vi "COMANDOS_QUIZ1.vi"() -> ()   [LabVIEW 2017]
panel:
  out "comentarios":string[](array[string])
  out "cmd users":string[](array[string])
  out "OP PRINCIPALES":T1(ring)
  out "CONFIG LED":T2(ring)
  out "CONFIG BOTON":T2(ring)
  out "L 3":string
  out "L 2":string
  out "L 1":string
  out "B 3":string
  out "B 2":string
  out "B 1":string
  out "time":u32
  out "contador":i32
  in  "TRAMA DE PRUEBA":string
  in  "BOTÓN 3":bool
  in  "BOTÓN 2":bool
  in  "BOTÓN 1":bool
  out "LED 3":bool
  out "LED 2":bool
  out "LED 1":bool
  out "at+<cmd>?response":string[](array[string])
  in  "stop":bool
  in  "send":bool
  out "Out":string
  in  "In":string
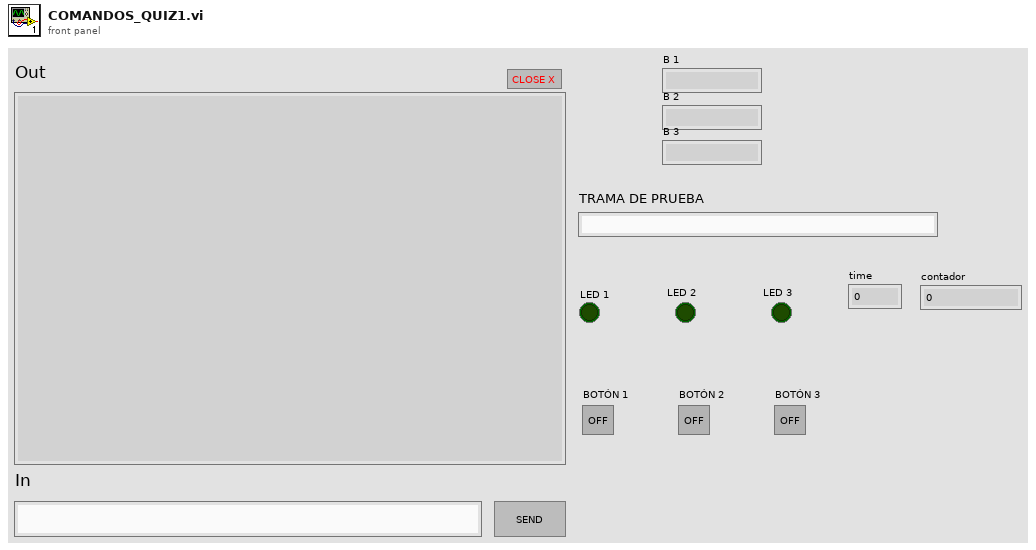
[diagram p1: front panel]
types:
  T1 = enum16{"AT", "AT+", "AT+HELP?", "AT+MAKE=", "AT+MAKE=?"}
  T2 = enum16{"ERROR", "1 ON", "1 OFF", "2 ON", "2 OFF", "3 ON", "3 OFF"}
  T3 = cluster{string, string, string, string, string, string, string, string, string, string, string, string, string, string, string, string}
  T4 = cluster{string, string, string, string, string, string}
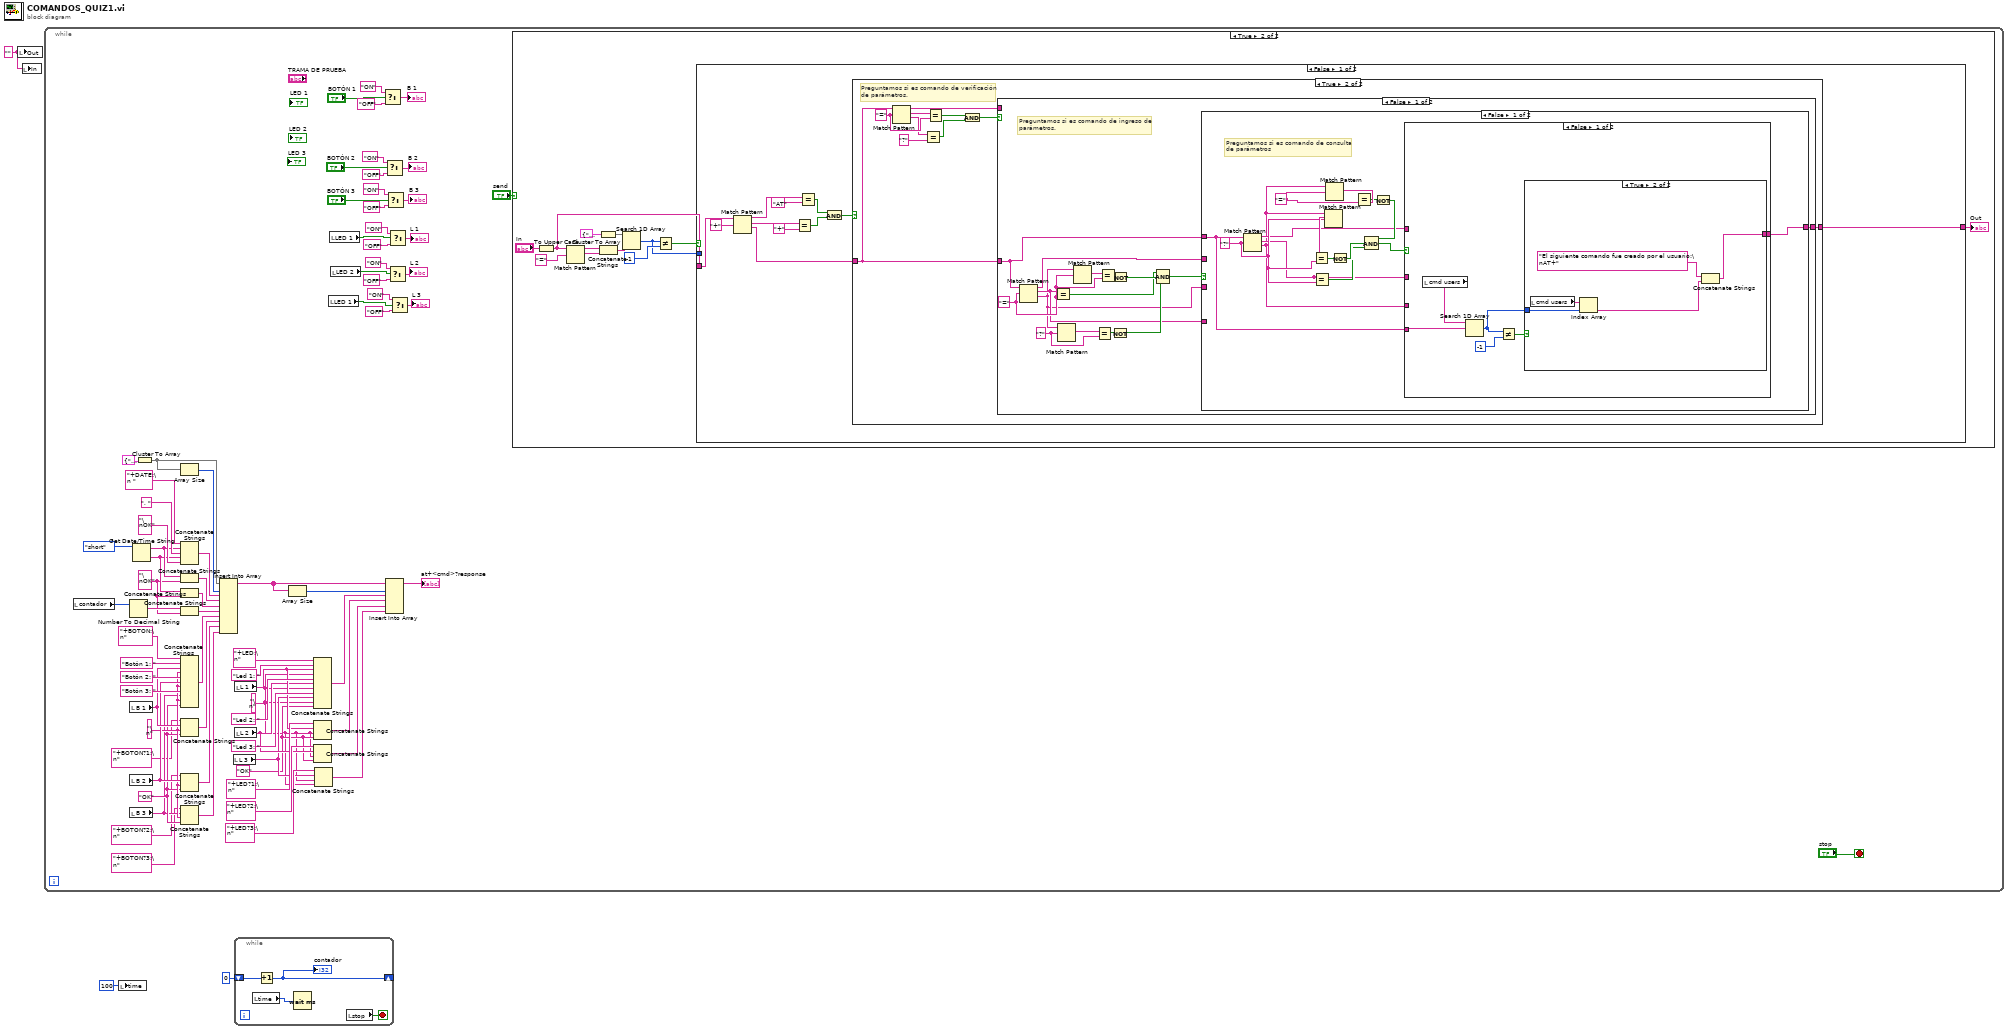
[diagram p0: block diagram]
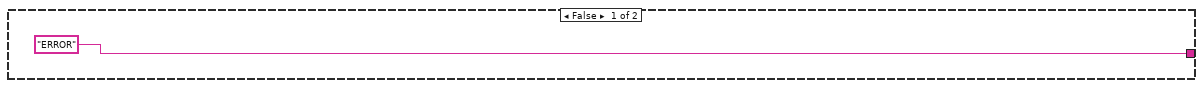
[diagram p3: hidden frame]
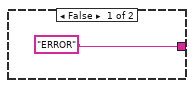
[diagram p4: hidden frame]
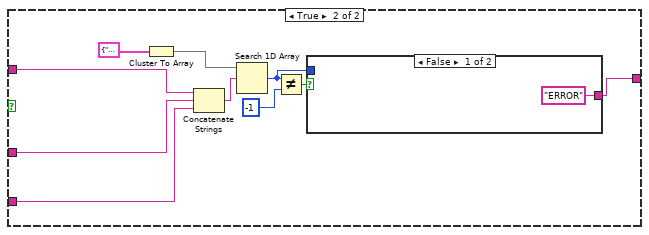
[diagram p5: hidden frame]
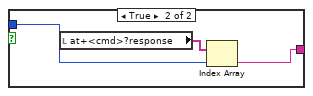
[diagram p6: hidden frame]
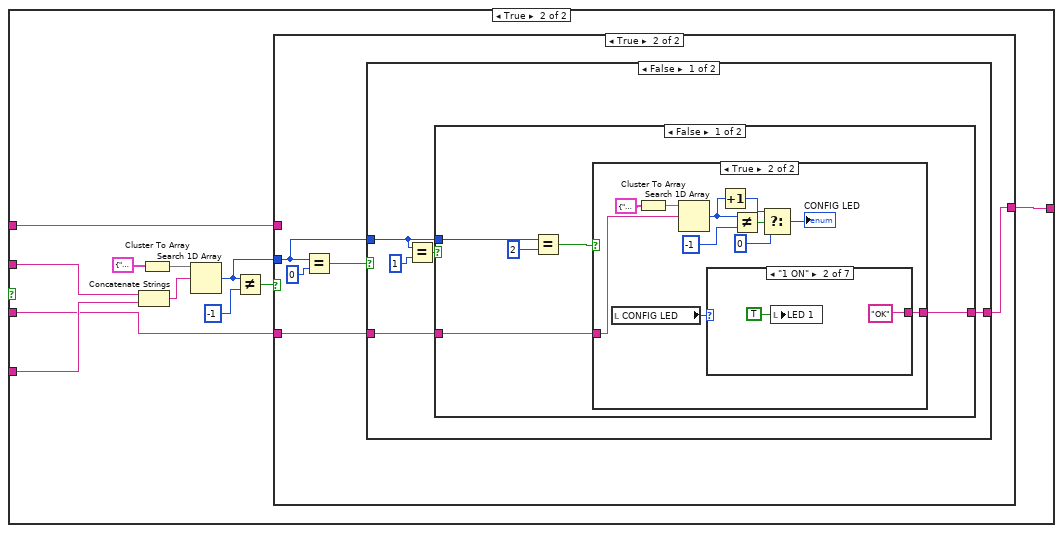
[diagram p7: hidden frame]
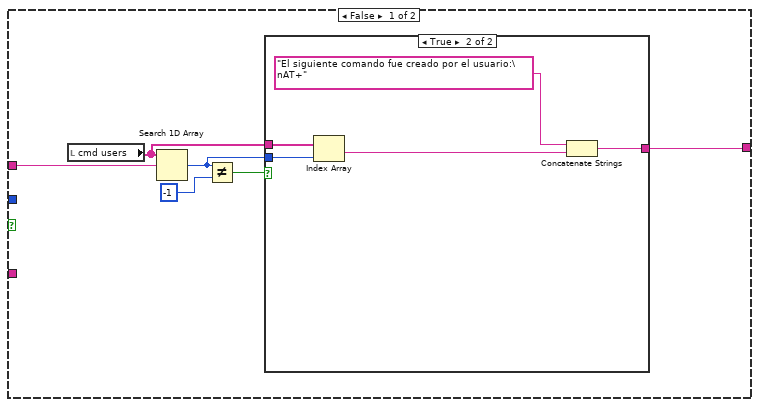
[diagram p8: hidden frame]
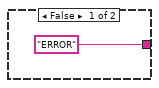
[diagram p9: hidden frame]
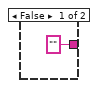
[diagram p10: hidden frame]
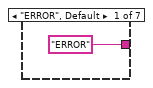
[diagram p11: hidden frame]
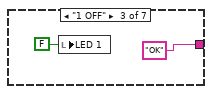
[diagram p12: hidden frame]
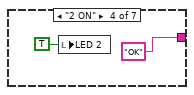
[diagram p13: hidden frame]
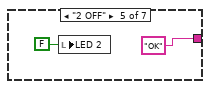
[diagram p14: hidden frame]
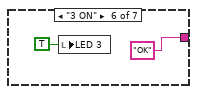
[diagram p15: hidden frame]
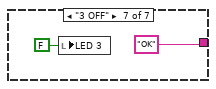
[diagram p16: hidden frame]
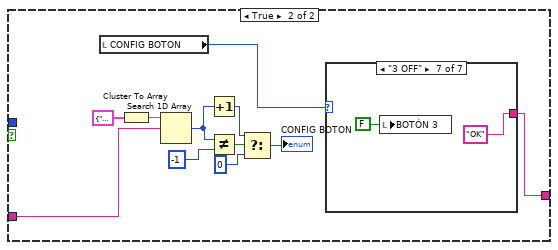
[diagram p17: hidden frame]
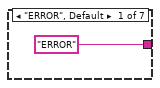
[diagram p18: hidden frame]
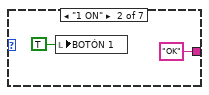
[diagram p19: hidden frame]
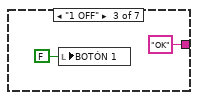
[diagram p20: hidden frame]
diagram:
  w3 = "" ("Out")
  n1 = local write "Out"(w3) -> ()
  n2 = local write "In"(w3) -> ()
  n3 = while {
    stop <- "stop" stop-if-true
    w12 = "OK" ("string")
    w11 = "\n" ("string")
    w42 = "OK" ("string")
    w43 = "\n" ("string")
    w65 = "\nOK" ("string")
    n4 = local read "contador"() -> (w67:i32)
    n5 = Number To Decimal String(number=w67) -> (decimal integer string=w66:string)  [unwired: 1 in]
    n6 = local read "B 1"() -> (w47:string)
    n7 = local read "B 2"() -> (w45:string)
    n8 = local read "B 3"() -> (w41:string)
    n9 = Get Date/Time String(date format (0)=enum16{"short", "long", "abbreviated"}."short") -> (date string=w72:string, time string=w71:string)  [unwired: 2 in]
    n10 = Cluster To Array(cluster=cluster{string, string, string, string} {"+GPS:\n$ GPRMC, 123519, A, 4807.038, N, 01131.000, E, 022.4,084.4,230394,003.1, W * 6A\n$ GPGGA, 123519,4807.038, N, 01131.000, E, 1,08,0.9,545.4, M, 46.9, M ,, * 47\n$ GPGSA, A, 3,04,05,, 09,12 ,,, 24 ,,,,, 2.5,1.3,2.1 * 39\nOK", "+GPS?RMC:\n$ GPRMC, 123519, A, 4807.038, N, 01131.000, E, 022.4,084.4,230394,003.1, W * 6A\nOK", "+GPS?GGA:\n$ GPGGA, 123519,4807.038, N, 01131.000, E, 1,08,0.9,545.4, M, 46.9, M ,, * 47\nOK", "+GPS?GSA:\n$ GPGSA, A, 3,04,05,, 09,12 ,,, 24 ,,,,, 2.5,1.3,2.1 * 39\nOK"}) -> (array=w74:string[])
    n11 = Array Size(array=w74) -> (size(s)=w76:i32)
    n12 = Concatenate Strings("+DATE:\n " ("string"), w72, ", " ("string"), w71, "\nOK" ("string")) -> (w70:string)
    n13 = Concatenate Strings(w72, w65) -> (w69:string)
    n14 = Concatenate Strings(w71, w65) -> (w68:string)
    n15 = Concatenate Strings(w66, w65) -> (w64:string)
    n16 = Concatenate Strings("+BOTON:\n" ("string"), "Botón 1: " ("string"), w47, w43, "Botón 2: " ("string"), w45, w43, "Botón 3: " ("string"), w41, w43, w42) -> (w48:string)
    n17 = Concatenate Strings("+BOTON?1:\n" ("string"), w47, w43, w42) -> (w46:string)
    n18 = Concatenate Strings("+BOTON?2:\n" ("string"), w45, w43, w42) -> (w44:string)
    n19 = Concatenate Strings("+BOTON?3:\n" ("string"), w41, w43, w42) -> (w40:string)
    n20 = Insert Into Array(array=w74, index=w76, new element #1=w70, new element #2=w69, new element #3=w68, new element #4=w64, new element #5=w48, new element #6=w46, new element #7=w44, new element #8=w40) -> (w6:string[])
    n21 = local read "L 3"() -> (w13:string)
    n22 = local read "L 1"() -> (w17:string)
    n23 = local read "L 2"() -> (w14:string)
    n24 = Array Size(array=w6) -> (size(s)=w5:i32)
    n25 = Concatenate Strings("+LED:\n" ("string"), "Led 1: " ("string"), w17, w11, "Led 2: " ("string"), w14, w11, "Led 3: " ("string"), w13, w11, w12) -> (w10:string)
    n26 = Concatenate Strings("+LED?1:\n" ("string"), w17, w11, w12) -> (w9:string)
    n27 = Concatenate Strings("+LED?2:\n" ("string"), w14, w11, w12) -> (w8:string)
    n28 = Concatenate Strings("+LED?3:\n" ("string"), w13, w11, w11) -> (w7:string)
    n29 = local read "LED 1"() -> (w28:bool)
    n30 = local read "LED 1"() -> (w36:bool)
    n31 = local read "LED 2"() -> (w35:bool)
    n32 = Select(t="ON", s="BOTÓN 1", f="OFF") -> (s? t:f=→"B 1":string)
    n33 = Insert Into Array(array=w6, index=w5, new element #1=w10, new element #2=w9, new element #3=w8, new element #4=w7) -> (→"at+<cmd>?response":string[])
    n34 = Select(t="ON", s="BOTÓN 2", f="OFF") -> (s? t:f=→"B 2":string)
    n35 = Select(t="ON", s="BOTÓN 3", f="OFF") -> (s? t:f=→"B 3":string)
    n36 = Select(t="ON", s=w35, f="OFF") -> (s? t:f=→"L 2":string)
    n37 = Select(t="ON", s=w36, f="OFF") -> (s? t:f=→"L 1":string)
    n38 = Select(t="ON", s=w28, f="OFF") -> (s? t:f=→"L 3":string)
    n39 = case shown="True" "send" {
      frame False {
      }
      frame True {
        n40 = To Upper Case(1:"In") -> (0:w85:string)
        n41 = Match Pattern(string=w85, regular expression="=") -> (before substring=w83:string, match substring=w82:string)  [unwired: 1 in, 2 out]
        n42 = Cluster To Array(cluster=cluster{string, string, string, string, string} {"AT", "AT+", "AT+HELP?", "AT+MAKE=", "AT+MAKE=?"}) -> (array=w90:string[])
        n43 = Concatenate Strings(w83, w82) -> (w81:string)
        n44 = Search 1D Array(1D array=w90, element=w81) -> (index of element=w86:i32)  [unwired: 1 in]
        n45 = Not Equal?(x=w86, y=-1) -> (x != y?=w88:bool)
        n46 = case shown="False" w88 {
          tunnel: w85 -> [w103 w291]
          tunnel: [w94 w292] -> w87
          tunnel: w86 -> [_ w294]
          frame False {
            n47 = Match Pattern(string=w103, regular expression="+") -> (before substring=w101:string, match substring=w98:string, after substring=w93:string)  [unwired: 1 in, 1 out]
            n48 = Equal?(x=w98, y="+") -> (x = y?=w97:bool)
            n49 = Equal?(x=w101, y="AT") -> (x = y?=w96:bool)
            n50 = And(x=w96, y=w97) -> (x .and. y?=w95:bool)
            n51 = case shown="True" w95 {
              tunnel: ["ERROR" w107] -> w94
              tunnel: w93 -> [_ w105]
              frame False {
              }
              frame True {
                w113 = "=" ("regular expression")
                # "Preguntamos si es comando de verificación\nde parámetros."
                n52 = Match Pattern(string=w105, regular expression=w113) -> (before substring=w108:string, match substring=w114:string, after substring=w112:string)  [unwired: 1 in, 1 out]
                n53 = Equal?(x=w112, y="?") -> (x = y?=w111:bool)
                n54 = Equal?(x=w114, y=w113) -> (x = y?=w110:bool)
                n55 = And(x=w110, y=w111) -> (x .and. y?=w109:bool)
                n56 = case shown="False" w109 {
                  tunnel: w108 -> [_ w267]
                  tunnel: [w119 w270] -> w107
                  tunnel: w105 -> [w118 w266]
                  frame False {
                    w126 = "?" ("regular expression")
                    w128 = "=" ("regular expression")
                    # "Preguntamos si es comando de ingreso de \nparámetros."
                    n57 = Match Pattern(string=w118, regular expression=w128) -> (before substring=w115:string, match substring=w117:string, after substring=w116:string)  [unwired: 1 in, 1 out]
                    n58 = Equal?(x=w117, y=w128) -> (x = y?=w121:bool)
                    n59 = Match Pattern(string=w116, regular expression=w126) -> (match substring=w127:string)  [unwired: 1 in, 3 out]
                    n60 = Match Pattern(string=w116, regular expression=w128) -> (match substring=w129:string)  [unwired: 1 in, 3 out]
                    n61 = Equal?(x=w127, y=w126) -> (x = y?=w124:bool)
                    n62 = Equal?(x=w129, y=w128) -> (x = y?=w125:bool)
                    n63 = Not(x=w124) -> (.not. x?=w122:bool)
                    n64 = Not(x=w125) -> (.not. x?=w123:bool)
                    n65 = Compound Arithmetic op=AND(w121, w123, w122) -> (w120:bool)
                    n66 = case shown="False" w120 {
                      tunnel: [w134 w174] -> w119
                      tunnel: w118 -> [w130 w171]
                      tunnel: w115 -> [_ w181]
                      tunnel: w117 -> [_ w180]
                      tunnel: w116 -> [_ w172]
                      frame False {
                        w143 = "=" ("regular expression")
                        w141 = "?" ("regular expression")
                        # "Preguntamos si es comando de consulta\nde parámetros"
                        n67 = Match Pattern(string=w130, regular expression=w141) -> (before substring=w133:string, match substring=w132:string, after substring=w131:string)  [unwired: 1 in, 1 out]
                        n68 = Equal?(x=w132, y=w141) -> (x = y?=w136:bool)
                        n69 = Match Pattern(string=w131, regular expression=w141) -> (match substring=w142:string)  [unwired: 1 in, 3 out]
                        n70 = Equal?(x=w142, y=w141) -> (x = y?=w139:bool)
                        n71 = Match Pattern(string=w131, regular expression=w143) -> (match substring=w144:string)  [unwired: 1 in, 3 out]
                        n72 = Not(x=w139) -> (.not. x?=w137:bool)
                        n73 = Equal?(x=w143, y=w144) -> (x = y?=w140:bool)
                        n74 = Not(x=w140) -> (.not. x?=w138:bool)
                        n75 = Compound Arithmetic op=AND(w138, w137, w136) -> (w135:bool)
                        n76 = case shown="False" w135 {
                          tunnel: [w146 w159] -> w134
                          tunnel: w133 -> [_ w165]
                          tunnel: w132 -> [_ w164]
                          tunnel: w131 -> [_ w158]
                          tunnel: w130 -> [w149 _]
                          frame False {
                            n77 = local read "cmd users"() -> (w150:string[])
                            n78 = Search 1D Array(1D array=w150, element=w149) -> (index of element=w145:i32)  [unwired: 1 in]
                            n79 = Not Equal?(x=w145, y=-1) -> (x != y?=w147:bool)
                            n80 = case shown="True" w147 {
                              tunnel: ["ERROR" w152] -> w146
                              tunnel: w145 -> [_ w155]
                              frame False {
                              }
                              frame True {
                                n81 = local read "cmd users"() -> (w156:string[])
                                n82 = Index Array(array=w156, index=w155) -> (element=w153:string)
                                n83 = Concatenate Strings("El siguiente comando fue creado por el usuario:\nAT+", w153) -> (w152:string)
                              }
                            }
                          }
                          frame True {
                            n84 = Cluster To Array(cluster=T3 {"GPS?", "GPS?RMC", "GPS?GGA", "GPS?GSA", "DATE?", "DATE?FECHA", "DATE?HORA", "COUNT?", "BOTON?", "BOTON?1", "BOTON?2", "BOTON?3", "LED?", "LED?1", "LED?2", "LED?3"}) -> (array=w157:string[])
                            n85 = Concatenate Strings(w165, w164, w158) -> (w163:string)
                            n86 = Search 1D Array(1D array=w157, element=w163) -> (index of element=w160:i32)  [unwired: 1 in]
                            n87 = Not Equal?(x=w160, y=-1) -> (x != y?=w161:bool)
                            n88 = case shown="False" w161 {
                              tunnel: w160 -> [_ w170]
                              tunnel: ["ERROR" w168] -> w159
                              frame False {
                              }
                              frame True {
                                n89 = local read "at+<cmd>?response"() -> (w169:string[])
                                n90 = Index Array(array=w169, index=w170) -> (element=w168:string)
                              }
                            }
                          }
                        }
                      }
                      frame True {
                        n91 = Concatenate Strings(w181, w180) -> (w177:string)
                        n92 = Cluster To Array(cluster=cluster{string, string, string} {"TIMECOUNT=", "BOTON=", "LED="}) -> (array=w178:string[])
                        n93 = Search 1D Array(1D array=w178, element=w177) -> (index of element=w173:i32)  [unwired: 1 in]
                        n94 = Not Equal?(x=w173, y=-1) -> (x != y?=w175:bool)
                        n95 = case shown="True" w175 {
                          tunnel: [w184 w195] -> w174
                          tunnel: w173 -> [_ w194]
                          tunnel: w172 -> [_ w196]
                          tunnel: w171 -> [w187 _]
                          frame False {
                            n96 = local read "cmd users"() -> (w183:string[])
                            n97 = Search 1D Array(1D array=w183, element=w187) -> (index of element=w182:i32)  [unwired: 1 in]
                            n98 = Not Equal?(x=w182, y=-1) -> (x != y?=w185:bool)
                            n99 = case shown="True" w185 {
                              tunnel: ["ERROR" w189] -> w184
                              tunnel: w183 -> [_ w193]
                              tunnel: w182 -> [_ w192]
                              frame False {
                              }
                              frame True {
                                n100 = Index Array(array=w193, index=w192) -> (element=w191:string)
                                n101 = Concatenate Strings("El siguiente comando fue creado por el usuario:\nAT+", w191) -> (w189:string)
                              }
                            }
                          }
                          frame True {
                            n102 = Equal?(x=w194, y=0) -> (x = y?=w197:bool)
                            n103 = case shown="False" w197 {
                              tunnel: w196 -> [w201 w265]
                              tunnel: [w200 w262] -> w195
                              tunnel: w194 -> [w199 _]
                              frame False {
                                n104 = Equal?(x=w199, y=1) -> (x = y?=w202:bool)
                                n105 = case shown="False" w202 {
                                tunnel: w201 -> [w205 w240]
                                tunnel: [w204 w234] -> w200
                                tunnel: w199 -> [w207 _]
                                frame False {
                                n106 = Equal?(x=w207, y=2) -> (x = y?=w206:bool)
                                n107 = case shown="True" w206 {
                                tunnel: w205 -> [_ w218]
                                tunnel: ["" w210] -> w204
                                frame False {
                                }
                                frame True {
                                n108 = local read "CONFIG LED"() -> (w211:T2)
                                n109 = Cluster To Array(cluster=T4 {"1,ON", "1,OFF", "2,ON", "2,OFF", "3,ON", "3,OFF"}) -> (array=w219:string[])
                                n110 = Search 1D Array(1D array=w219, element=w218) -> (index of element=w215:i32)  [unwired: 1 in]
                                n111 = case shown="\"1 ON\"" w211 {
                                tunnel: ["ERROR" "OK" "OK" "OK" "OK" "OK" "OK"] -> w210
                                frame "ERROR", Default {
                                }
                                frame "1 ON" {
                                n112 = local write "LED 1"(TRUE ("LED 1")) -> ()
                                }
                                frame "1 OFF" {
                                n113 = local write "LED 1"(FALSE ("LED 1")) -> ()
                                }
                                frame "2 ON" {
                                n114 = local write "LED 2"(TRUE ("LED 1")) -> ()
                                }
                                frame "2 OFF" {
                                n115 = local write "LED 2"(FALSE ("LED 1")) -> ()
                                }
                                frame "3 ON" {
                                n116 = local write "LED 3"(TRUE ("LED 1")) -> ()
                                }
                                frame "3 OFF" {
                                n117 = local write "LED 3"(FALSE ("LED 1")) -> ()
                                }
                                }
                                n118 = Increment(x=w215) -> (x+1=w214:i32)
                                n119 = Not Equal?(x=w215, y=-1) -> (x != y?=w216:bool)
                                n120 = Select(t=w214, s=w216, f=0) -> (s? t:f=→"CONFIG LED":i32)
                                }
                                }
                                }
                                frame True {
                                n121 = local read "CONFIG BOTON"() -> (w235:T2)
                                n122 = Cluster To Array(cluster=T4 {"1,ON", "1,OFF", "2,ON", "2,OFF", "3,ON", "3,OFF"}) -> (array=w243:string[])
                                n123 = Search 1D Array(1D array=w243, element=w240) -> (index of element=w239:i32)  [unwired: 1 in]
                                n124 = Increment(x=w239) -> (x+1=w238:i32)
                                n125 = Not Equal?(x=w239, y=-1) -> (x != y?=w241:bool)
                                n126 = Select(t=w238, s=w241, f=0) -> (s? t:f=→"CONFIG BOTON":i32)
                                n127 = case shown="\"3 OFF\"" w235 {
                                tunnel: ["ERROR" "OK" "OK" "OK" "OK" "OK" "OK"] -> w234
                                frame "ERROR", Default {
                                }
                                frame "1 ON" {
                                n128 = local write "BOTÓN 1"(TRUE ("BOTÓN 1")) -> ()
                                }
                                frame "1 OFF" {
                                n129 = local write "BOTÓN 1"(FALSE ("BOTÓN 1")) -> ()
                                }
                                frame "2 ON" {
                                n130 = local write "BOTÓN 2"(TRUE ("BOTÓN 1")) -> ()
                                }
                                frame "2 OFF" {
                                n131 = local write "BOTÓN 2"(FALSE ("BOTÓN 1")) -> ()
                                }
                                frame "3 ON" {
                                n132 = local write "BOTÓN 3"(TRUE ("BOTÓN 1")) -> ()
                                }
                                frame "3 OFF" {
                                n133 = local write "BOTÓN 3"(FALSE ("BOTÓN 1")) -> ()
                                }
                                }
                                }
                                }
                              }
                              frame True {
                                n134 = Decimal String To Number(string=w265) -> (number=w260:i32)  [unwired: 2 in, 1 out]
                                n135 = Equal To 0?(x=w260) -> (x = 0?=w261:bool)
                                n136 = Select(t="ERROR ", s=w261, f="OK ") -> (s? t:f=w262:string)
                                n137 = Select(t=100, s=w261, f=w260) -> (s? t:f=→"time":i32)
                              }
                            }
                          }
                        }
                      }
                    }
                  }
                  frame True {
                    w269 = cluster{string, string, string} {"TIMECOUNT", "BOTON", "LED"}  # at<cmd>=?
                    n138 = Cluster To Array(cluster=w269) -> (array=w268:string[])
                    n139 = Search 1D Array(1D array=w268, element=w267) -> (index of element=w271:i32)  [unwired: 1 in]
                    n140 = Not Equal?(x=w271, y=-1) -> (x != y?=w272:bool)
                    n141 = case shown="False" w272 {
                      tunnel: w271 -> [_ w290]
                      tunnel: [w275 w289] -> w270
                      tunnel: w266 -> [w274 _]
                      frame False {
                        n142 = local read "cmd users"() -> (w278:string[])
                        n143 = Search 1D Array(1D array=w278, element=w274) -> (index of element=w276:i32)  [unwired: 1 in]
                        n144 = Not Equal?(x=w276, y=-1) -> (x != y?=w277:bool)
                        n145 = case shown="True" w277 {
                          tunnel: w276 -> [_ w285]
                          tunnel: ["ERROR" w282] -> w275
                          frame False {
                          }
                          frame True {
                            n146 = local read "cmd users"() -> (w286:string[])
                            n147 = Index Array(array=w286, index=w285) -> (element=w283:string)
                            n148 = Concatenate Strings("El siguiente comando fue creado por el usuario:\n", w283, "\nOK" ("string")) -> (w282:string)
                          }
                        }
                      }
                      frame True {
                        w287 = cluster{string, string, string} {"at+timecount=?\n+timecount: (tiempo en milisegundos)", "at+boton=?\n+boton: (id pulsador),(estado)", "at+led=?\n+led: (id led),(estado)"}  # at<cmd>=?response
                        n149 = Cluster To Array(cluster=w287) -> (array=w288:string[])
                        n150 = Index Array(array=w288, index=w290) -> (element=w289:string)
                      }
                    }
                  }
                }
              }
            }
          }
          frame True {
            n151 = local read "OP PRINCIPALES"() -> (w293:T1)
            n152 = case shown="\"AT+MAKE=?\"" w293 {
              tunnel: ["OK" "OK" "LISTA DE COMANDOS:\nAT: comando de prueba.\nAT+: comando de prueba.\nAT+HELP?: muestra la lista de comandos.\nAT+MAKE=: crea un comando.\nAT+MAKE=?: muestra prototipo para crear comando.\nAT+GPS?: muestra las tramas gps.\nAT+GPS?RMC: muestra la trama rmc.\nAT+GPS?GGA: muestra la trama gga.\nAT+GPS?GSA: muestra la trama gsa.\nAT+DATE?: muestra la fecha y hora del sistema.\nAT+DATE?FECHA: muestra la fecha del sistema.\nAT+DATE?HORA:  muestra la hora del sistema.\nAT+TIMECOUNT=: muestra el tiempo de actualización del contador.\nAT+TIMECOUNT=? muestra el prototio de la función timecount.\nAT+COUNT?: muestra el valor del contador.\nAT+BOTON=: asigna un estado a alguno de los botones.\nAT+BOTON=?: muestra el prototipo de la función boton.\nAT+BOTON?: muestra el estado de los bototes\nAT+BOTON?1: muestra el estado del botón 1\nAT+BOTON?2: muestra el estado del botón 2\nAT+BOTON?3: muestra el estado del botón 3\nAT+LED=:asigna un estado a alguno de los led\nAT+LED=?: muestra el prototipo de la función led.\nAT+LED?: muestra el estado de los leds.\nAT+LED?1: muestra el estado del led 1.\nAT+LED?2: muestra el estado del led 2.\nAT+LED?3: muestra el estado del led 3.\n\n\n\n\n\n" w302 "+MAKE=?:\nAT+MAKE=(CMD),(COMENTARIO)\nOK"] -> w292
              tunnel: w291 -> [_ _ _ w308 _]
              frame "AT", Default {
              }
              frame "AT+" {
              }
              frame "AT+HELP?" {
              }
              frame "AT+MAKE=" {
                w304 = ",\"" ("regular expression")
                n153 = Match Pattern(string=w308, regular expression="=") -> (after substring=w306:string)  [unwired: 1 in, 3 out]
                n154 = Match Pattern(string=w306, regular expression=w304) -> (before substring=w301:string, match substring=w305:string, after substring=w300:string)  [unwired: 1 in, 1 out]
                n155 = Equal?(x=w305, y=w304) -> (x = y?=w303:bool)
                n156 = Match Pattern(string=w300, regular expression="\"") -> (before substring=w298:string)  [unwired: 1 in, 3 out]
                n157 = case shown="True" w303 {
                  tunnel: ["ERROR" w313] -> w302
                  tunnel: w301 -> [_ w321]
                  tunnel: w298 -> [_ w310]
                  frame False {
                  }
                  frame True {
                    n158 = Match Pattern(string=w321, regular expression="+") -> (before substring=w311:string, match substring=w318:string, after substring=w312:string)  [unwired: 1 in, 1 out]
                    n159 = Equal?(x=w318, y="+") -> (x = y?=w315:bool)
                    n160 = Equal?(x=w311, y="AT") -> (x = y?=w316:bool)
                    n161 = And(x=w316, y=w315) -> (x .and. y?=w314:bool)
                    n162 = case shown="True" w314 {
                      tunnel: ["ERROR" w336] -> w313
                      tunnel: w312 -> [_ w324]
                      tunnel: w310 -> [_ w323]
                      frame False {
                      }
                      frame True {
                        w330 = "=" ("regular expression")
                        n163 = Match Pattern(string=w324, regular expression=w330) -> (before substring=w332:string, match substring=w335:string, after substring=w334:string)  [unwired: 1 in, 1 out]
                        n164 = Equal?(x=w335, y=w330) -> (x = y?=w328:bool)
                        n165 = Equal?(x=w334, y="?") -> (x = y?=w327:bool)
                        n166 = Equal?(x=w332, y="") -> (x = y?=w329:bool)
                        n167 = Not(x=w329) -> (.not. x?=w325:bool)
                        n168 = Compound Arithmetic op=AND(w325, w328, w327) -> (w326:bool)
                        n169 = case shown="True" w326 {
                          tunnel: [w339 "OK"] -> w336
                          tunnel: w324 -> [w338 w383]
                          tunnel: w323 -> [w337 w379]
                          frame False {
                            w346 = "?" ("regular expression")
                            n170 = Match Pattern(string=w338, regular expression=w346) -> (before substring=w350:string, match substring=w347:string, after substring=w345:string)  [unwired: 1 in, 1 out]
                            n171 = Equal?(x=w350, y="") -> (x = y?=w348:bool)
                            n172 = Equal?(x=w345, y="") -> (x = y?=w341:bool)
                            n173 = Equal?(x=w347, y=w346) -> (x = y?=w342:bool)
                            n174 = Not(x=w348) -> (.not. x?=w343:bool)
                            n175 = Compound Arithmetic op=AND(w343, w342, w341) -> (w340:bool)
                            n176 = case shown="True" w340 {
                              tunnel: [w353 "OK"] -> w339
                              tunnel: w338 -> [w352 w376]
                              tunnel: w337 -> [w351 w373]
                              frame False {
                                w358 = "=" ("regular expression")
                                n177 = Match Pattern(string=w352, regular expression=w358) -> (before substring=w363:string, match substring=w359:string, after substring=w361:string)  [unwired: 1 in, 1 out]
                                n178 = Not Equal?(x=w363, y="") -> (x != y?=w357:bool)
                                n179 = Equal?(x=w359, y=w358) -> (x = y?=w356:bool)
                                n180 = Not Equal?(x=w361, y="") -> (x != y?=w355:bool)
                                n181 = Compound Arithmetic op=AND(w357, w356, w355) -> (w354:bool)
                                n182 = case shown="True" w354 {
                                tunnel: ["ERROR" "OK"] -> w353
                                tunnel: w352 -> [_ w369]
                                tunnel: w351 -> [_ w366]
                                frame False {
                                }
                                frame True {
                                n183 = local read "comentarios"() -> (w367:string[])
                                n184 = local read "cmd users"() -> (w370:string[])
                                n185 = Build Array (concatenate)(w367, w366) -> (w365:string[])
                                n186 = Build Array (concatenate)(w370, w369) -> (w368:string[])
                                n187 = local write "comentarios"(w365) -> ()
                                n188 = local write "cmd users"(w368) -> ()
                                }
                                }
                              }
                              frame True {
                                n189 = local read "comentarios"() -> (w374:string[])
                                n190 = local read "cmd users"() -> (w377:string[])
                                n191 = Build Array (concatenate)(w377, w376) -> (w375:string[])
                                n192 = Build Array (concatenate)(w374, w373) -> (w372:string[])
                                n193 = local write "cmd users"(w375) -> ()
                                n194 = local write "comentarios"(w372) -> ()
                              }
                            }
                          }
                          frame True {
                            n195 = local read "comentarios"() -> (w380:string[])
                            n196 = local read "cmd users"() -> (w384:string[])
                            n197 = Build Array (concatenate)(w380, w379) -> (→"comentarios":string[])
                            n198 = Build Array (concatenate)(w384, w383) -> (→"cmd users":string[])
                          }
                        }
                      }
                    }
                  }
                }
              }
              frame "AT+MAKE=?" {
              }
            }
            "OP PRINCIPALES" <- w294
          }
        }
        "Out" <- w87
      }
    }
  }
  n199 = local write "time"(u32 100 ("time")) -> ()
  n200 = while {
    shift-right: [w389] -> _
    shift-left: 0 -> [w388]
    stop <- w390 stop-if-true
    n201 = local read "time"() -> (w387:u32)
    n202 = Increment(x=w388) -> (x+1=w389:i32)
    "contador" <- w389
    n203 = Wait (ms)(milliseconds to wait=w387) -> ()  [unwired: 1 out]
    n204 = local read "stop"() -> (w390:bool)
  }
